vi "Select AcquireParams to Display.vi"(1 "ACQUIPARAMS":T2 {"CFA"."CFA" items=["CFA_NONE", "CFA_VRI", "CFA_VRIV6", "CFA_BAYER", "CFA_BAYERFLIP"]; "TriggerTime"."fractions" format="%32.0f"}) -> (0 "ACQUIPARAMS Display":T1)   [LabVIEW 2013, in "VRI.lvlib"]
uses:
  VRI.lvlib
  _Type Defs/Rect.ctl
  _Type Defs/PHCon Time64.ctl
  _Type Defs/PHCon ACQUIPARAMS.ctl
  _Type Defs/PhInt CFA.ctl
  _Type Defs/PhCon SyncImaging.ctl
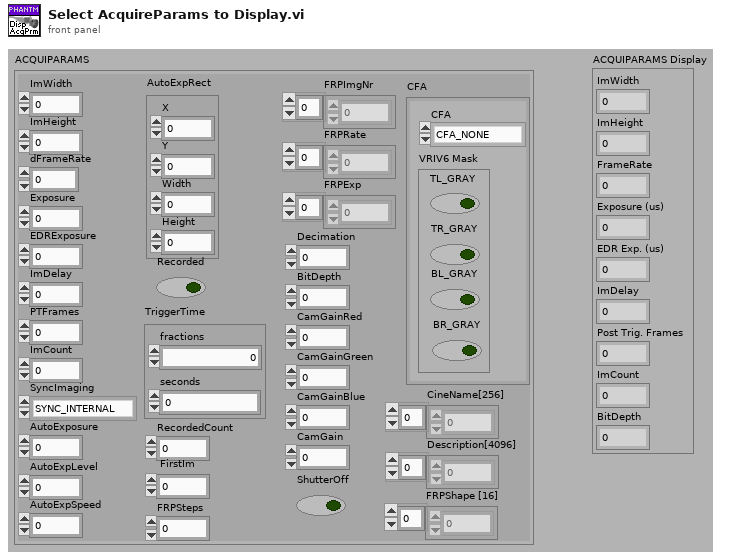
[diagram p1: front panel]
types:
  T1 = cluster{"ImWidth":u32, "ImHeight":u32, "FrameRate":u32, "Exposure (us)":u32, "EDR Exp. (us)":u32, "ImDelay":u32, "Post Trig. Frames":u32, "ImCount":u32, "BitDepth":u32}
  T2 = typedef "VRI.lvlib/PHCon ACQUIPARAMS.ctl" = cluster{"ImWidth":u32, "ImHeight":u32, "(deprecated)FrameRateInt":u32, "Exposure":u32, "EDRExposure":u32, "ImDelay":u32, "PTFrames":u32, "ImCount":u32, "SyncImaging":T3, "AutoExposure":u32, "AutoExpLevel":u32, "AutoExpSpeed":u32, "AutoExpRect":T4, "Recorded":bool, "TriggerTime":T5, "RecordedCount":u32, "FirstIm":i32, "FRPSteps":u32, "FRPImgNr":i32[], "FRPRate":u32[], "FRPExp":u32[], "Decimation":u32, "BitDepth":u32, "CamGainRed":u32, "CamGainGreen":u32, "CamGainBlue":u32, "CamGain":u32, "ShutterOff":bool, "CFA":T6, "CineName[256]":u8[], "Description[4096]":u8[], "FRPShape [16]":u32[], "dFrameRate":dbl}
  T3 = typedef "VRI.lvlib/PhCon SyncImaging.ctl" = enum32{"SYNC_INTERNAL", "SYNC_EXTERNAL", "SYNC_LOCKTOIRIG"}
  T4 = typedef "VRI.lvlib/Rect.ctl" = cluster{"X":i32, "Y":i32, "Width":i32, "Height":i32}
  T5 = typedef "VRI.lvlib/PHCon Time64.ctl" = cluster{"fractions":u32, "seconds":u32}
  T6 = typedef "VRI.lvlib/PhInt CFA.ctl" = cluster{"CFA":u32, "VRIV6 Mask":cluster{"TL_GRAY":bool, "TR_GRAY":bool, "BL_GRAY":bool, "BR_GRAY":bool}}
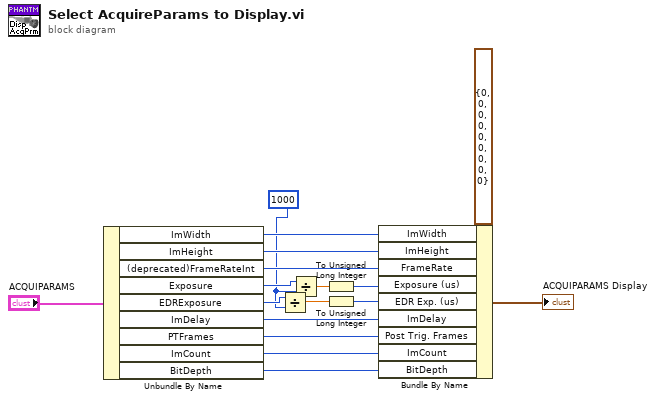
[diagram p0: block diagram]
diagram:
  w4 = u32 1000 ("y")
  n1 = Unbundle By Name("ACQUIPARAMS") -> ("ImWidth"=w15:u32, "ImHeight"=w14:u32, "(deprecated)FrameRateInt"=w13:u32, "Exposure"=w6:u32, "EDRExposure"=w5:u32, "ImDelay"=w12:u32, "PTFrames"=w11:u32, "ImCount"=w10:u32, "BitDepth"=w9:u32)
  n2 = Divide(x=w5, y=w4) -> (x/y=w3:dbl)
  n3 = Divide(x=w6, y=w4) -> (x/y=w7:dbl)
  n4 = To Unsigned Long Integer(number=w7) -> (unsigned 32bit integer=w1:u32)
  n5 = To Unsigned Long Integer(number=w3) -> (unsigned 32bit integer=w2:u32)
  n6 = Bundle By Name(cluster=T1 {"ImWidth"=0, "ImHeight"=0, "FrameRate"=0, "Exposure (us)"=0, "EDR Exp. (us)"=0, "ImDelay"=0, "Post Trig. Frames"=0, "ImCount"=0, "BitDepth"=0} ("ACQUIPARAMS Display"), "ImWidth"=w15, "ImHeight"=w14, "FrameRate"=w13, "Exposure (us)"=w1, "EDR Exp. (us)"=w2, "ImDelay"=w12, "Post Trig. Frames"=w11, "ImCount"=w10, "BitDepth"=w9) -> (→"ACQUIPARAMS Display":T1)
